vi "KrakenSetVoltageComp.vi"(0 "DeviceReference (in)":T2, 5 "Set Voltage Compensation Mode":bool, 9 "DeviceConfiguration (in)":T1={"Future Proof Configs"=FALSE, "MotorOutputInverted"=0, "MotorOutputNeutralMode"=0, "MotorOutputDutyCycleNeutralDeadband"=0.0, "MotorOutputPeakForwardDutyCycle"=1.0, "MotorOutputPeakReverseDutyCycle"=-1.0, "CurrentLimitsStatorCurrentLimit"=0.0, "CurrentLimitsStatorCurrentLimitEnable"=FALSE, "CurrentLimitsSupplyCurrentLimit"=0.0, "CurrentLimitsSupplyCurrentLimitEnable"=FALSE, "CurrentLimitsSupplyCurrentThreshold"=0.0, "CurrentLimitsSupplyTimeThreshold"=0.0, "VoltageSupplyVoltageTimeConstant"=0.0, "VoltagePeakForwardVoltage"=16.0, "VoltagePeakReverseVoltage"=-16.0, "TorqueCurrentPeakForwardTorqueCurrent"=800.0, "TorqueCurrentPeakReverseTorqueCurrent"=-800.0, "TorqueCurrentTorqueNeutralDeadband"=0.0, "FeedbackFeedbackRotorOffset"=0.0, "FeedbackSensorToMechanismRatio"=1.0, "FeedbackRotorToSensorRatio"=1.0, "FeedbackFeedbackSensorSource"=0, "FeedbackFeedbackRemoteSensorID"=0, "DifferentialSensorsDifferentialSensorSource"=0, "DifferentialSensorsDifferentialTalonFXSensorID"=0, "DifferentialSensorsDifferentialRemoteSensorID"=0, "DifferentialConstantsPeakDifferentialDutyCycle"=2.0, "DifferentialConstantsPeakDifferentialVoltage"=32.0, "DifferentialConstantsPeakDifferentialTorqueCurrent"=1600.0, "OpenLoopRampsDutyCycleOpenLoopRampPeriod"=0.0, "OpenLoopRampsVoltageOpenLoopRampPeriod"=0.0, "OpenLoopRampsTorqueOpenLoopRampPeriod"=0.0, "ClosedLoopRampsDutyCycleClosedLoopRampPeriod"=0.0, "ClosedLoopRampsVoltageClosedLoopRampPeriod"=0.0, "ClosedLoopRampsTorqueClosedLoopRampPeriod"=0.0, "HardwareLimitSwitchForwardLimitType"=0, "HardwareLimitSwitchForwardLimitAutosetPositionEnable"=FALSE, "HardwareLimitSwitchForwardLimitAutosetPositionValue"=0.0, "HardwareLimitSwitchForwardLimitEnable"=TRUE, "HardwareLimitSwitchForwardLimitSource"=0, "HardwareLimitSwitchForwardLimitRemoteSensorID"=0, "HardwareLimitSwitchReverseLimitType"=0, "HardwareLimitSwitchReverseLimitAutosetPositionEnable"=FALSE, "HardwareLimitSwitchReverseLimitAutosetPositionValue"=0.0, "HardwareLimitSwitchReverseLimitEnable"=TRUE, "HardwareLimitSwitchReverseLimitSource"=0, "HardwareLimitSwitchReverseLimitRemoteSensorID"=0, "AudioBeepOnBoot"=TRUE, "AudioBeepOnConfig"=TRUE, "AudioAllowMusicDurDisable"=FALSE, "SoftwareLimitSwitchForwardSoftLimitEnable"=FALSE, "SoftwareLimitSwitchReverseSoftLimitEnable"=FALSE, "SoftwareLimitSwitchForwardSoftLimitThreshold"=0.0, "SoftwareLimitSwitchReverseSoftLimitThreshold"=0.0, "MotionMagicMotionMagicCruiseVelocity"=0.0, "MotionMagicMotionMagicAcceleration"=0.0, "MotionMagicMotionMagicJerk"=0.0, "MotionMagicMotionMagicExpo_kV"=0.0, "MotionMagicMotionMagicExpo_kA"=0.0, "CustomParamsCustomParam0"=0, "CustomParamsCustomParam1"=0, "ClosedLoopGeneralContinuousWrap"=FALSE, "Slot0kP"=0.0, "Slot0kI"=0.0, "Slot0kD"=0.0, "Slot0kS"=0.0, "Slot0kV"=0.0, "Slot0kA"=0.0, "Slot0kG"=0.0, "Slot0GravityType"=0, "Slot0StaticFeedforwardSign"=0, "Slot1kP"=0.0, "Slot1kI"=0.0, "Slot1kD"=0.0, "Slot1kS"=0.0, "Slot1kV"=0.0, "Slot1kA"=0.0, "Slot1kG"=0.0, "Slot1GravityType"=0, "Slot1StaticFeedforwardSign"=0, "Slot2kP"=0.0, "Slot2kI"=0.0, "Slot2kD"=0.0, "Slot2kS"=0.0, "Slot2kV"=0.0, "Slot2kA"=0.0, "Slot2kG"=0.0, "Slot2GravityType"=0, "Slot2StaticFeedforwardSign"=0} {"MotorOutputInverted" items=["CounterClockwise_Positive", "Clockwise_Positive"]; "MotorOutputNeutralMode" items=["Coast", "Brake"]; "FeedbackFeedbackSensorSource" items=["RotorSensor", "RemoteCANcoder", "RemotePigeon2_Yaw", "RemotePigeon2_Pitch", "RemotePigeon2_Roll", "FusedCANcoder", "SyncCANcoder"]; "DifferentialSensorsDifferentialSensorSource" items=["Disabled", "RemoteTalonFX_Diff", "RemotePigeon2_Yaw", "RemotePigeon2_Pitch", "RemotePigeon2_Roll", "RemoteCANcoder"]; "HardwareLimitSwitchForwardLimitType" items=["NormallyOpen", "NormallyClosed"]; "HardwareLimitSwitchForwardLimitSource" items=["LimitSwitchPin"=0, "RemoteTalonFX"=1, "RemoteCANifier"=2, "RemoteCANcoder"=4, "Disabled"=3]; "HardwareLimitSwitchReverseLimitType" items=["NormallyOpen", "NormallyClosed"]; "HardwareLimitSwitchReverseLimitSource" items=["LimitSwitchPin"=0, "RemoteTalonFX"=1, "RemoteCANifier"=2, "RemoteCANcoder"=4, "Disabled"=3]; "Slot0GravityType" items=["Elevator_Static", "Arm_Cosine"]; "Slot0StaticFeedforwardSign" items=["UseVelocitySign", "UseClosedLoopSign"]; "Slot1GravityType" items=["Elevator_Static", "Arm_Cosine"]; "Slot1StaticFeedforwardSign" items=["UseVelocitySign", "UseClosedLoopSign"]; "Slot2GravityType" items=["Elevator_Static", "Arm_Cosine"]; "Slot2StaticFeedforwardSign" items=["UseVelocitySign", "UseClosedLoopSign"]}, 11 "Error (in)":errorcluster) -> (4 "DeviceReference (out)":T2, 10 "DeviceConfiguration (out)":T1, 15 "Error (out)":errorcluster)   [LabVIEW 2023]
doc: "Wrapper for setting voltage compensation mode for Talon FX motor controllers."
uses:
  3ee01901-79ae-4aa6-af32-efcf4cf19248.vi
  <vilib>/Rock Robotics/WPI/ThirdParty/Phoenix6/DeviceReference.ctl
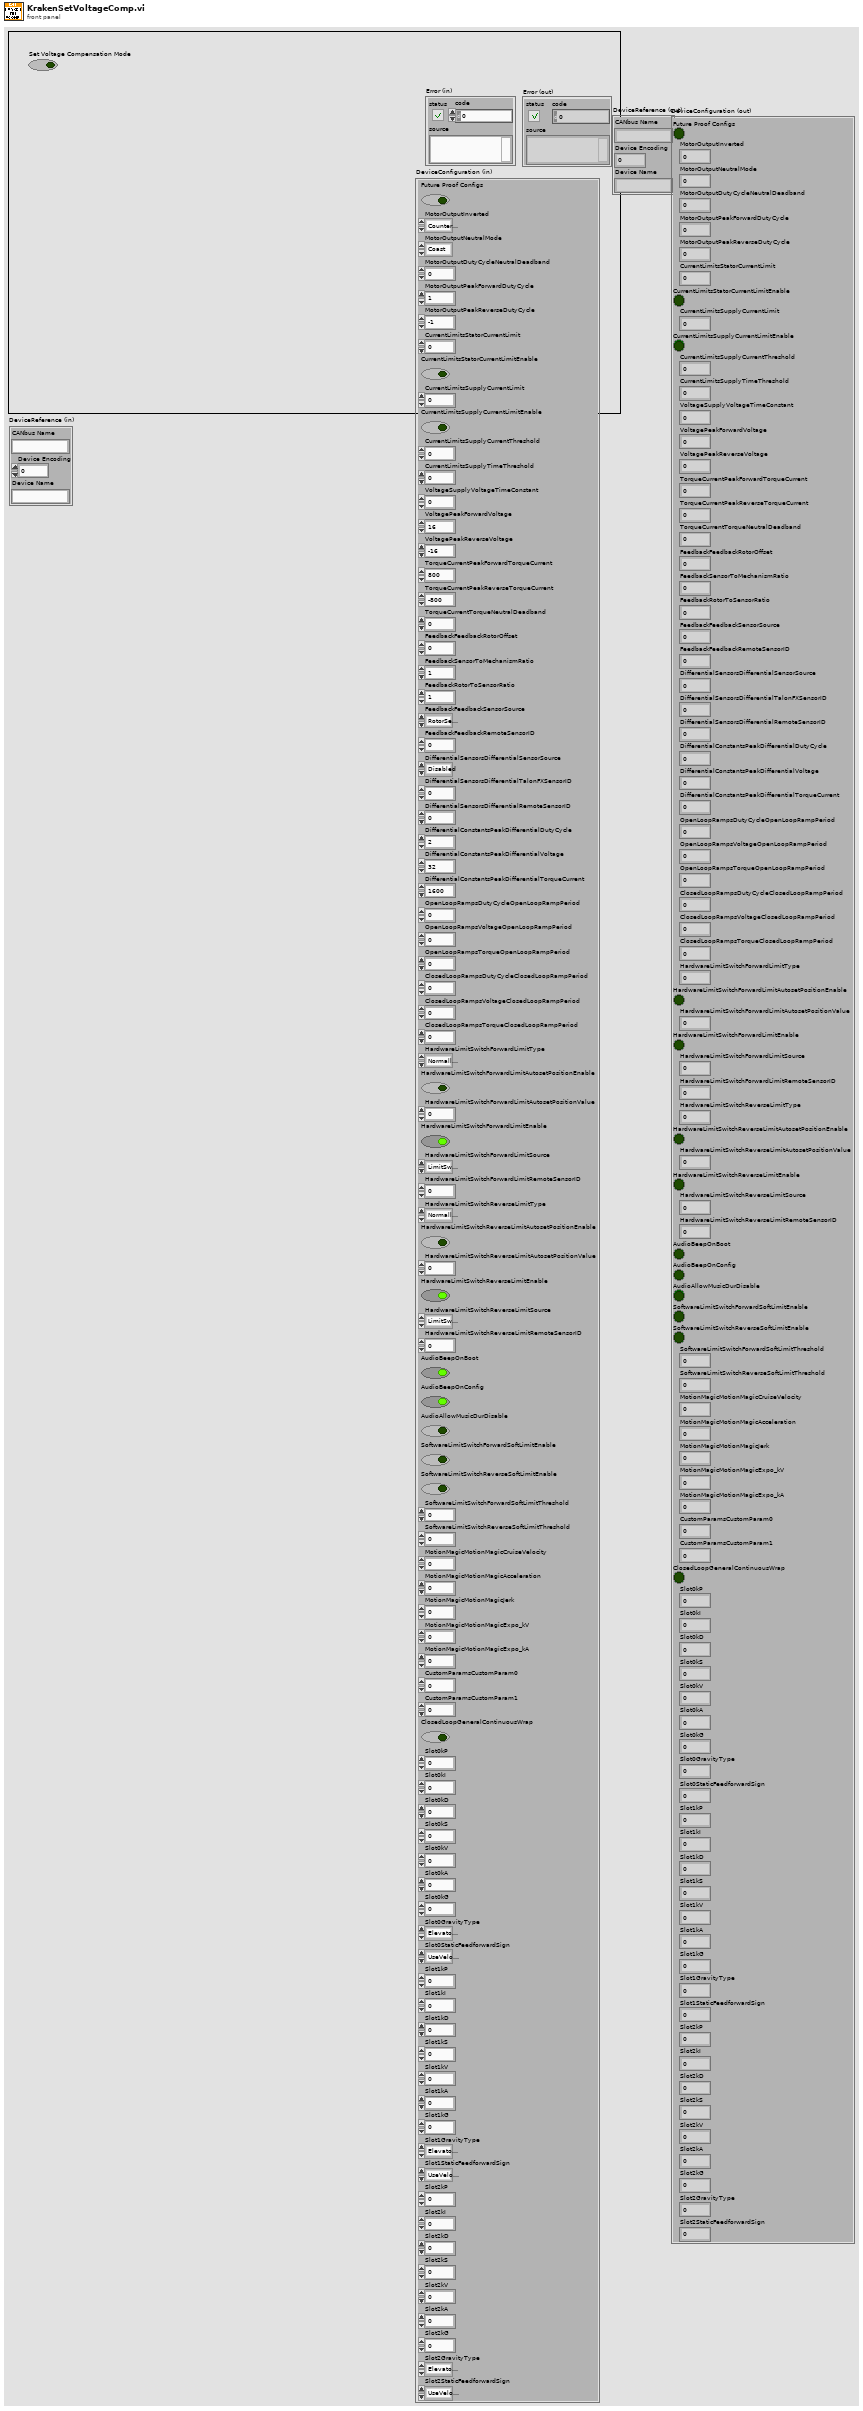
[diagram p1: front panel]
types:
  T1 = cluster{"Future Proof Configs":bool, "MotorOutputInverted":u16, "MotorOutputNeutralMode":u16, "MotorOutputDutyCycleNeutralDeadband":dbl, "MotorOutputPeakForwardDutyCycle":dbl, "MotorOutputPeakReverseDutyCycle":dbl, "CurrentLimitsStatorCurrentLimit":dbl, "CurrentLimitsStatorCurrentLimitEnable":bool, "CurrentLimitsSupplyCurrentLimit":dbl, "CurrentLimitsSupplyCurrentLimitEnable":bool, "CurrentLimitsSupplyCurrentThreshold":dbl, "CurrentLimitsSupplyTimeThreshold":dbl, "VoltageSupplyVoltageTimeConstant":dbl, "VoltagePeakForwardVoltage":dbl, "VoltagePeakReverseVoltage":dbl, "TorqueCurrentPeakForwardTorqueCurrent":dbl, "TorqueCurrentPeakReverseTorqueCurrent":dbl, "TorqueCurrentTorqueNeutralDeadband":dbl, "FeedbackFeedbackRotorOffset":dbl, "FeedbackSensorToMechanismRatio":dbl, "FeedbackRotorToSensorRatio":dbl, "FeedbackFeedbackSensorSource":u16, "FeedbackFeedbackRemoteSensorID":i16, "DifferentialSensorsDifferentialSensorSource":u16, "DifferentialSensorsDifferentialTalonFXSensorID":i16, "DifferentialSensorsDifferentialRemoteSensorID":i16, "DifferentialConstantsPeakDifferentialDutyCycle":dbl, "DifferentialConstantsPeakDifferentialVoltage":dbl, "DifferentialConstantsPeakDifferentialTorqueCurrent":dbl, "OpenLoopRampsDutyCycleOpenLoopRampPeriod":dbl, "OpenLoopRampsVoltageOpenLoopRampPeriod":dbl, "OpenLoopRampsTorqueOpenLoopRampPeriod":dbl, "ClosedLoopRampsDutyCycleClosedLoopRampPeriod":dbl, "ClosedLoopRampsVoltageClosedLoopRampPeriod":dbl, "ClosedLoopRampsTorqueClosedLoopRampPeriod":dbl, "HardwareLimitSwitchForwardLimitType":u16, "HardwareLimitSwitchForwardLimitAutosetPositionEnable":bool, "HardwareLimitSwitchForwardLimitAutosetPositionValue":dbl, "HardwareLimitSwitchForwardLimitEnable":bool, "HardwareLimitSwitchForwardLimitSource":u16, "HardwareLimitSwitchForwardLimitRemoteSensorID":i16, "HardwareLimitSwitchReverseLimitType":u16, "HardwareLimitSwitchReverseLimitAutosetPositionEnable":bool, "HardwareLimitSwitchReverseLimitAutosetPositionValue":dbl, "HardwareLimitSwitchReverseLimitEnable":bool, "HardwareLimitSwitchReverseLimitSource":u16, "HardwareLimitSwitchReverseLimitRemoteSensorID":i16, "AudioBeepOnBoot":bool, "AudioBeepOnConfig":bool, "AudioAllowMusicDurDisable":bool, "SoftwareLimitSwitchForwardSoftLimitEnable":bool, "SoftwareLimitSwitchReverseSoftLimitEnable":bool, "SoftwareLimitSwitchForwardSoftLimitThreshold":dbl, "SoftwareLimitSwitchReverseSoftLimitThreshold":dbl, "MotionMagicMotionMagicCruiseVelocity":dbl, "MotionMagicMotionMagicAcceleration":dbl, "MotionMagicMotionMagicJerk":dbl, "MotionMagicMotionMagicExpo_kV":dbl, "MotionMagicMotionMagicExpo_kA":dbl, "CustomParamsCustomParam0":i16, "CustomParamsCustomParam1":i16, "ClosedLoopGeneralContinuousWrap":bool, "Slot0kP":dbl, "Slot0kI":dbl, "Slot0kD":dbl, "Slot0kS":dbl, "Slot0kV":dbl, "Slot0kA":dbl, "Slot0kG":dbl, "Slot0GravityType":u16, "Slot0StaticFeedforwardSign":u16, "Slot1kP":dbl, "Slot1kI":dbl, "Slot1kD":dbl, "Slot1kS":dbl, "Slot1kV":dbl, "Slot1kA":dbl, "Slot1kG":dbl, "Slot1GravityType":u16, "Slot1StaticFeedforwardSign":u16, "Slot2kP":dbl, "Slot2kI":dbl, "Slot2kD":dbl, "Slot2kS":dbl, "Slot2kV":dbl, "Slot2kA":dbl, "Slot2kG":dbl, "Slot2GravityType":u16, "Slot2StaticFeedforwardSign":u16}
  T2 = typedef "DeviceReference.ctl" = cluster{"CANbus Name":string, "Device Encoding":u32, "Device Name":string}
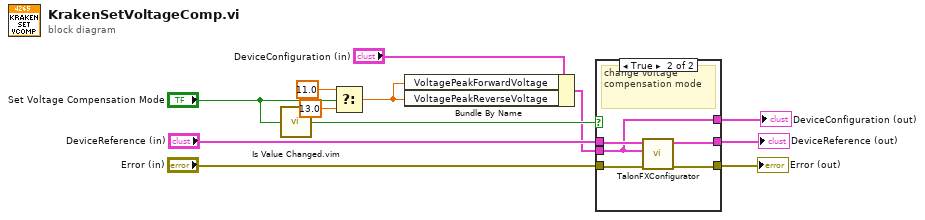
[diagram p0: block diagram]
diagram:
  n1 = call "Is Value Changed.vim"("value"="Set Voltage Compensation Mode") -> ("changed or first call?"=w11:bool)
  n2 = Select(t=11.0, s="Set Voltage Compensation Mode", f=13.0) -> (s? t:f=w4:dbl)
  n3 = Bundle By Name(cluster="DeviceConfiguration (in)", "VoltagePeakForwardVoltage"=w4, "VoltagePeakReverseVoltage"=w4) -> (w3:T1)
  n4 = case shown="True" w11 {
    tunnel: "DeviceReference (in)" -> [w15 w17]
    tunnel: [w15 w17] -> w2
    tunnel: "Error (in)" -> [w14 w18]
    tunnel: [w14 w19] -> w10
    tunnel: w3 -> [w13 w16]
    tunnel: [w13 w16] -> w1
    frame False {
    }
    frame True {
      # "change voltage compensation mode"
      n5 = call <vilib>:"TalonFXConfigurator.vi"("error in"=w18, "DeviceConfiguration"=w16, "DeviceReference"=w17) -> ("error out"=w19:errorcluster)  [unwired: 8 in]
    }
  }
  "Error (out)" <- w10
  "DeviceReference (out)" <- w2
  "DeviceConfiguration (out)" <- w1
